vi "Connect.vi"(8 "error in (no error)":errorcluster, 9 "timeout in ms (10000)":i32=10000, 11 "Communication in":refnum<class "Network.lvclass">) -> (0 "error out":errorcluster, 3 "Communication out":refnum<class "Network.lvclass">)   [LabVIEW 2020, in "Communication Classes.lvlib" / "Network.lvclass"]
uses:
  Network.lvclass
  IP_Communication/IP_Communication.lvclass
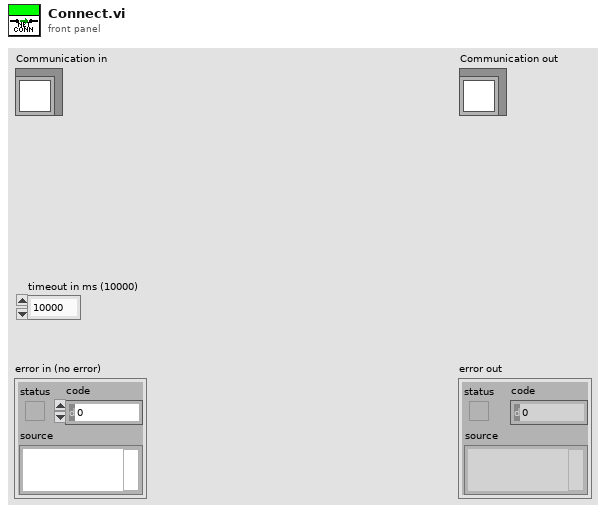
[diagram p1: front panel]
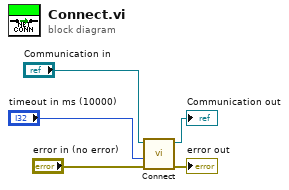
[diagram p0: block diagram]
diagram:
  n1 = call-parent "Connect.vi"("error in (no error)"="error in (no error)", "timeout in ms (10000)"="timeout in ms (10000)", "Communication in"="Communication in") -> ("error out"=→"error out":errorcluster, "Communication out"=→"Communication out":refnum<class "Network.lvclass">)  [unwired: 7 in]
